vi "message box enable.vi"() -> ()   [LabVIEW 2016]
panel:
  in  "enable":bool
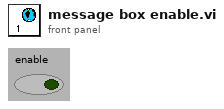
[diagram p1: front panel]
diagram:
